vi "Test no error 1097.vi"() -> ()   [LabVIEW 2013, in "libssh2_tests.lvlib"]
uses:
  libssh2_tests.lvlib
  libssh2/libssh2_init_default.vi
  <vilib>/addons/_JKI Toolkits/Caraya/classes/Assert/Assert Equal Value_Variant.vi
  <vilib>/addons/_JKI Toolkits/Caraya/classes/Assert/Assert Not Equal Value_Variant.vi
  libssh2/libssh2.lvlib
  <vilib>/addons/_JKI Toolkits/Caraya/classes/Assert/Assert.lvclass
  <vilib>/addons/_JKI Toolkits/Caraya/classes/Test/Test.lvclass
panel:
  out "error out":errorcluster
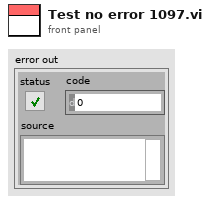
[diagram p1: front panel]
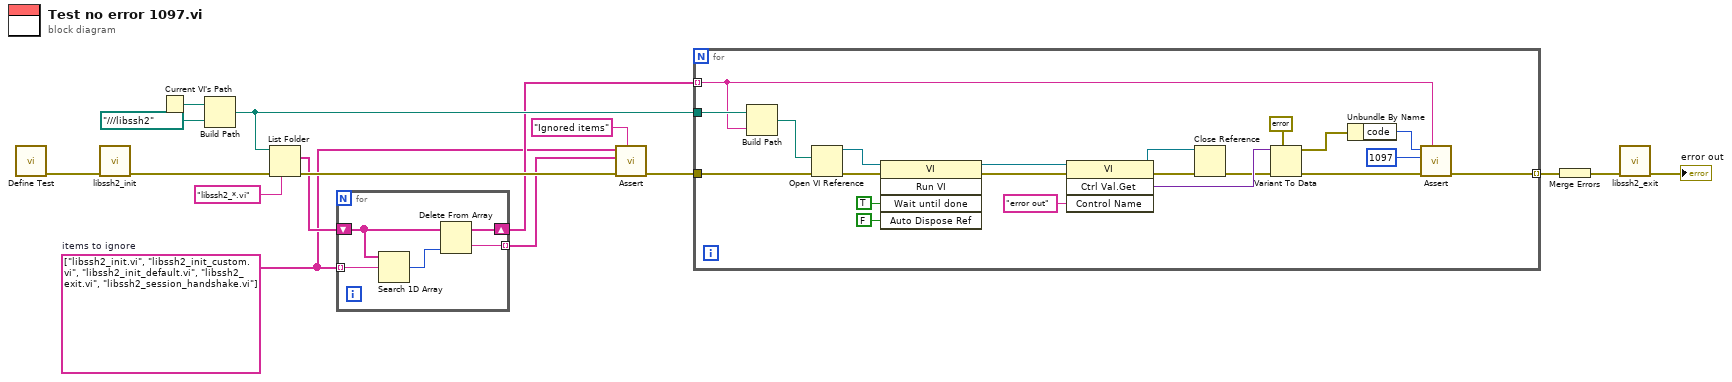
[diagram p0: block diagram]
diagram:
  w3 = string[] ["libssh2_init.vi", "libssh2_init_custom.vi", "libssh2_init_default.vi", "libssh2_exit.vi", "libssh2_session_handshake.vi"]  # items to ignore
  n1 = call <vilib>:"Define Test.vi"() -> ("error out"=w11:errorcluster)  [unwired: 10 in, 1 out]
  n2 = call-poly "libssh2_init.vi"("error in (no error)"=w11) -> ("error out"=w9:errorcluster)  [unwired: 10 in]
  n3 = Current VI's Path() -> (path=w16:path)
  n4 = Build Path(base path=w16, name or relative path=path "../../../libssh2" ("base path")) -> (appended path=w13:path)
  n5 = List Folder(path=w13, pattern="libssh2_*.vi", error in=w9) -> (filenames=w6:string[], error out=w10:errorcluster)  [unwired: 1 in, 2 out]
  n6 = for {
    shift-right: [w19] -> w5
    shift-left: w6 -> [w20]
    tunnel: w3 -> [w21] mode=indexing
    tunnel: [w17] -> w2 mode=indexing
    n7 = Search 1D Array(1D array=w20, element=w21) -> (index of element=w18:i32)  [unwired: 1 in]
    n8 = Delete From Array(array=w20, index=w18) -> (deleted portion=w17:string, array with subset deleted=w19:string[])  [unwired: 1 in]
  }
  n9 = call-poly <vilib>:"Assert.vi"("Label"="Ignored items", "error in (no error)"=w10, "Y"=w2, "X"=w3) -> ("error out"=w4:errorcluster)  [unwired: 6 in, 1 out]
  n10 = for {
    tunnel: w13 -> [w42]
    tunnel: [w23] -> w12 mode=indexing
    tunnel: w4 -> [w30]
    tunnel: w5 -> [w25] mode=indexing
    n11 = Build Path(base path=w42, name or relative path=w25) -> (appended path=w41:path)
    n12 = Open VI Reference(vi path=w41, error in (no error)=w30) -> (vi reference=w40:refnum<vi>, error out=w36:errorcluster)  [unwired: 4 in]
    n13 = invoke on="Invoke Node" class="VI" method="Run VI"(reference=w40, error in=w36, "Wait until done"=TRUE ("Wait Until Done"), "Auto Dispose Ref"=FALSE ("Auto Dispose Reference")) -> (reference out=w39:refnum<vi>, error out=w35:errorcluster)  [unwired: 1 in, 3 out]
    n14 = invoke on="Invoke Node" class="VI" method="Ctrl Val.Get"(reference=w39, error in=w35, "Control Name"="error out") -> (reference out=w28:refnum<vi>, error out=w33:errorcluster, "Get Control Value Variant"=w32:variant)  [unwired: 1 in, 1 out]
    n15 = Close Reference(reference=w28, error in (no error)=w33) -> (error out=w29:errorcluster)
    n16 = Variant To Data(error in=w29, type=errorcluster {"status"=FALSE, "code"=0, "source"=""} ("error in (no error)"), Variant=w32) -> (data=w22:errorcluster, error out=w24:errorcluster)
    n17 = Unbundle By Name(w22) -> ("code"=w27:i32)
    n18 = call-poly <vilib>:"Assert.vi"("Label"=w25, "error in (no error)"=w24, "Y"=1097 ("code"), "X"=w27) -> ("error out"=w23:errorcluster)  [unwired: 6 in, 1 out]
  }
  n19 = Merge Errors(w12) -> (w7:errorcluster)
  n20 = call "libssh2_exit.vi"("error in (no error)"=w7) -> ("error out"=→"error out":errorcluster)  [unwired: 10 in]
